vi "get FPGA resource reservation info.vi"(8 "error in (no error)":errorcluster, 10 "Name in Bitfile":string, 11 "Item Ref in":T1 format="%.0x") -> (0 "error out":errorcluster, 1 "found?":bool, 2 "Reserver Node Ref":T1=18446744073709551615 format="%.0x", 3 "Item Ref out":T1 format="%.0x", 4 "notes":string)   [LabVIEW 2016, in "FPGA Resource Manager.lvlib"]
uses:
  FPGA Resource Manager.lvlib
  <vilib>/NI Veristand/Custom Device API/Custom Device Item Ref.ctl
  <vilib>/NI Veristand/Custom Device API/Get Item Property (String).vi
  <vilib>/NI Veristand/Custom Device API/Get Item Property (Dependent Node Pointer).vi
  <vilib>/NI VeriStand/Custom Device API/Custom Device API.lvlib
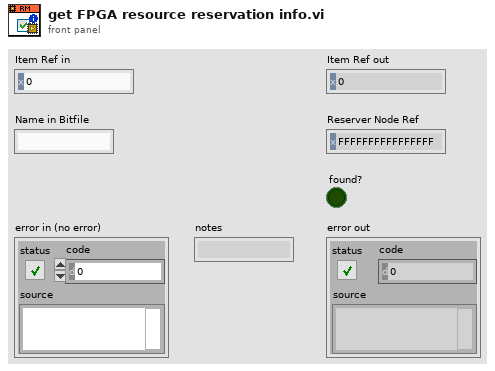
[diagram p1: front panel]
types:
  T1 = typedef "Custom Device API.lvlib/Custom Device Item Ref.ctl" = u64
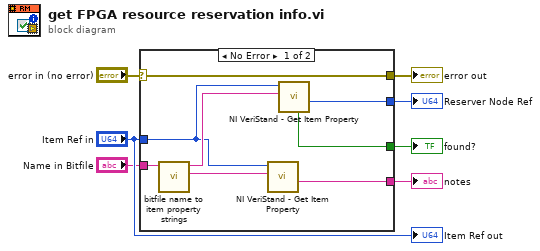
[diagram p0: block diagram]
diagram:
  n1 = case shown="No Error" "error in (no error)" {
    selector: "error in (no error)" -> [w15 w16]
    tunnel: [w15 w16] -> w6
    tunnel: "Item Ref in" -> [w9 _]
    tunnel: "Name in Bitfile" -> [w12 _]
    tunnel: [w14 _] -> w4
    tunnel: [w13 _] -> w3
    tunnel: [w8 _] -> w1
    frame No Error {
      n2 = call "bitfile name to item property strings.vi"("Name in bitfile"=w12) -> ("Notes String"=w10:string, "Reservation String"=w11:string)  [unwired: 9 in]
      n3 = call-poly <vilib>:"NI VeriStand - Get Item Property.vi"("Property Name"=w10, "Item Ref in"=w9) -> ("Value"=w8:string)  [unwired: 6 in, 3 out]
      n4 = call-poly <vilib>:"NI VeriStand - Get Item Property.vi"("Property Name"=w11, "Item Ref in"=w9) -> ("Dependent Node Ref"=w13:T1, "Found"=w14:bool)  [unwired: 6 in, 2 out]
    }
    frame Error {
    }
  }
  "error out" <- w6
  "found?" <- w4
  "Reserver Node Ref" <- w3
  "notes" <- w1
  "Item Ref out" <- "Item Ref in"
